vi "Send command to AutoCAD.vi"(4 "File name suffix":string, 5 "DesignRequest":T2, 6 "AC Variables":string[](array[string]), 7 "Mathcad Output":T3, 8 "error in (no error)":errorcluster, 9 "progress":refnum<vi>, 10 "Add":refnum<k24>, 11 "AutoCad app in":refnum<k24>) -> (0 "error out":errorcluster, 1 "progress out":refnum<vi>, 2 "Add out":refnum<k24>, 3 "AutoCad app out":refnum<k24>)   [LabVIEW 2012, in "Design Server.lvlib"]
uses:
  Design Server.lvlib
  Variable cluster.ctl
  Design Request.ctl
  C:/Program Files/Autodesk/AutoCAD 2013/Autodesk.AutoCAD.Interop.dll
  Program Files/Autodesk/AutoCAD 2013/Autodesk.AutoCAD.Interop.dll
panel:
  out "timing":T1
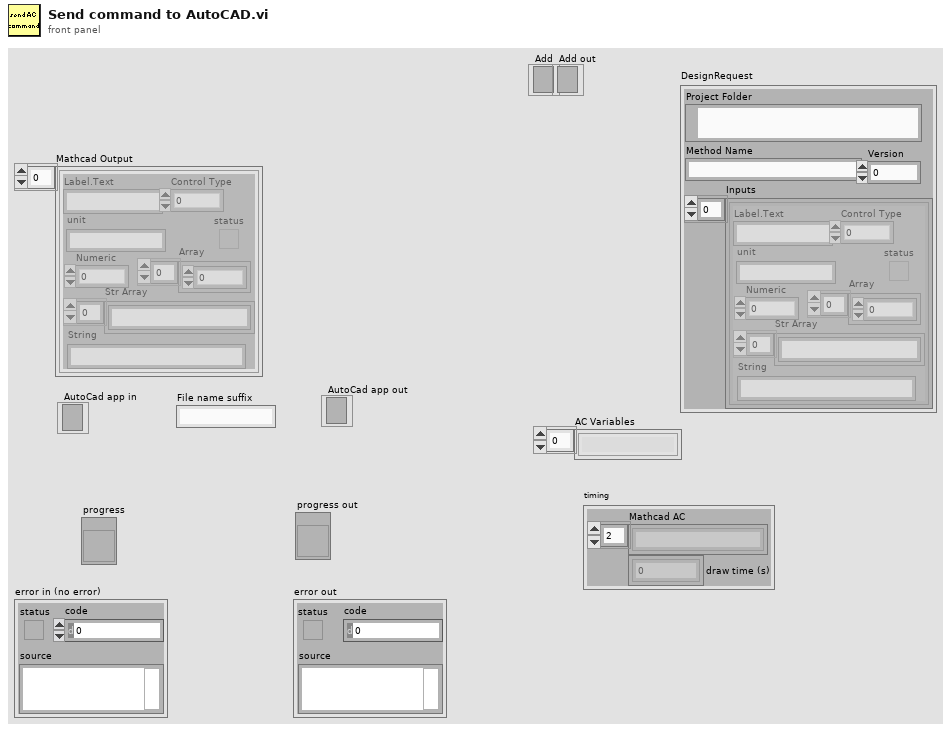
[diagram p1: front panel]
types:
  T1 = cluster{"draw time (s)":dbl[], "Mathcad AC":string[]}
  T2 = typedef "Design Server.lvlib/Design Request.ctl" = cluster{"Project Folder":path, "Method Name":string, "Inputs":T3, "Version":i32}
  T3 = typedef "Design Server.lvlib/Variable cluster.ctl" = cluster{"Label.Text":string, "Control Type":u32, "Numeric":dbl, "Array":dbl[], "status":bool, "Str Array":string[], "String":string, "unit":string}[]
  T4 = enum16{"open", "replace", "create", "open or create", "replace or create", "replace or create with confirmation"}
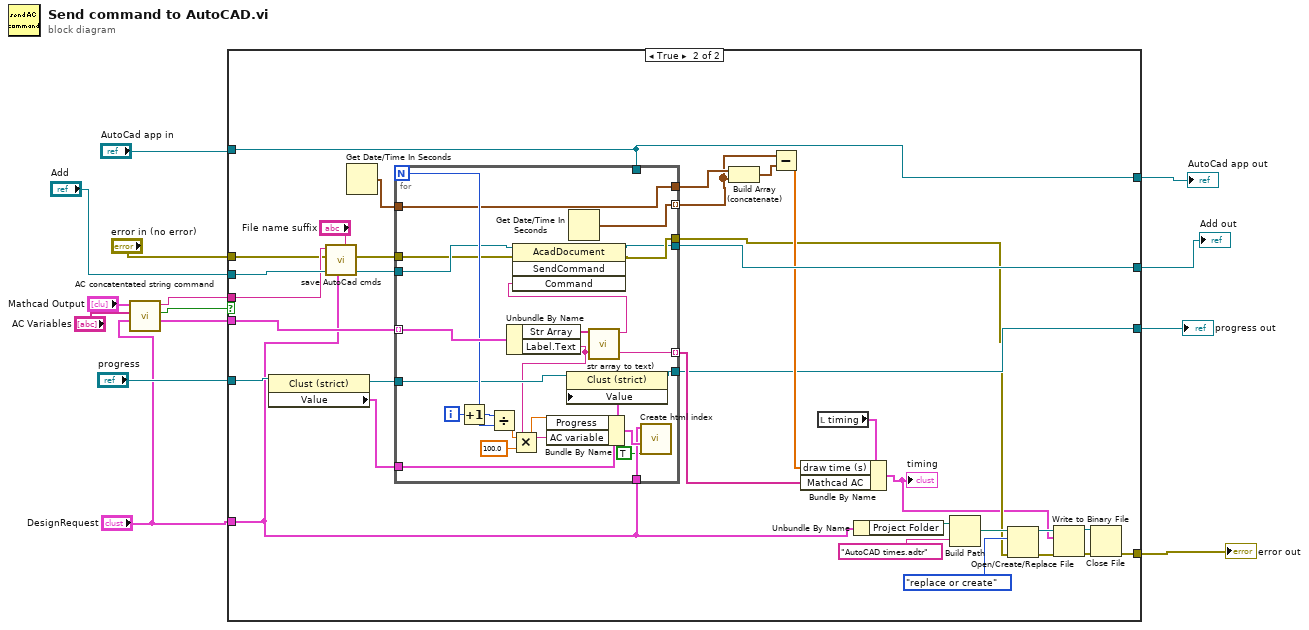
[diagram p0: block diagram]
diagram:
  n1 = call "AC concatentated string command.vi"("DesignRequest"="DesignRequest", "AC Variables"="AC Variables", "MathCAD results"="Mathcad Output") -> ("MathCAD AC"=w14:T3, "Has AC commands"=w8:bool, "AC concatenated string"=w6:string)  [unwired: 6 in]
  n2 = case shown="True" w8 {
    tunnel: w14 -> [_ w24]
    tunnel: [w18 w19] -> w3
    tunnel: "AutoCad app in" -> [w18 w19]
    tunnel: [w16 w48] -> w1
    tunnel: "Add" -> [w16 w47]
    tunnel: "error in (no error)" -> [w17 w21]
    tunnel: [w17 w34] -> w11
    tunnel: "progress" -> [w15 w30]
    tunnel: [w15 w29] -> w9
    tunnel: w6 -> [_ w25]
    tunnel: "DesignRequest" -> [_ w20]
    frame False {
    }
    frame True {
      n3 = property class="Clust (strict)"(reference=w30) -> (reference out=w49:refnum<vi>, "Value"=w42:cluster{"Progress":u8, "AC variable":string})  [unwired: 1 in, 1 out]
      n4 = call "save AutoCad cmds.vi"("File name suffix"="File name suffix", "DesignRequest"=w20, "error in"=w21, "AC.txt"=w25) -> ("error out"=w22:errorcluster)  [unwired: 7 in]
      n5 = Get Date/Time In Seconds() -> (seconds since 1Jan1904=w45:timestamp)
      n6 = for {
        N -> [w66]
        tunnel: w22 -> [w53]
        tunnel: w24 -> [w71] mode=indexing
        tunnel: w47 -> [w54]
        tunnel: [w50] -> w48
        tunnel: [w51] -> w28
        tunnel: w19 -> [_]
        tunnel: w49 -> [w61]
        tunnel: w42 -> [w70]
        tunnel: [w68] -> w29
        tunnel: [w55] -> w44 mode=indexing
        tunnel: [w60] -> w46
        tunnel: w45 -> [w60]
        tunnel: [w59] -> w40 mode=indexing
        tunnel: w20 -> [w57]
        i -> [w67]
        n7 = Increment(x=w67) -> (x+1=w62:i32)
        n8 = Divide(x=w62, y=w66) -> (x/y=w65:dbl)
        n9 = Unbundle By Name(w71) -> ("Str Array"=w69:string[], "Label.Text"=w59:string)
        n10 = Multiply(x=w65, y=100.0) -> (x*y=w63:dbl)
        n11 = Bundle By Name(cluster=w70, "Progress"=w63, "AC variable"=w59) -> (w58:cluster{"Progress":u8, "AC variable":string})
        n12 = property class="Clust (strict)"(reference=w61, "Value"=w58) -> (reference out=w68:refnum<vi>)  [unwired: 1 in, 1 out]
        n13 = Get Date/Time In Seconds() -> (seconds since 1Jan1904=w55:timestamp)
        n14 = call "str array to text).vi"("Array"=w69) -> ("String"=w52:string)  [unwired: 10 in]
        n15 = invoke class="AcadDocument" method="SendCommand"(reference=w54, error in=w53, "Command"=w52) -> (reference out=w50:refnum<k24>, error out=w51:errorcluster)  [unwired: 1 in, 2 out]
        n16 = call "Create html index.vi"("progress"=w58, "Under construction"=TRUE, "DesignRequest"=w57) -> ()  [unwired: 7 in, 2 out]
      }
      n17 = Build Array (concatenate)(w46, w44) -> (w43:timestamp[])
      n18 = Subtract(x=w44, y=w43) -> (x-y=w41:dbl[])
      n19 = local read "timing"() -> (w27:T1)
      n20 = Bundle By Name(cluster=w27, "draw time (s)"=w41, "Mathcad AC"=w40) -> (w26:T1)
      "timing" <- w26
      n21 = Unbundle By Name(w20) -> ("Project Folder"=w33:path)
      n22 = Build Path(base path=w33, name or relative path="AutoCAD times.adtr") -> (appended path=w31:path)
      n23 = Open/Create/Replace File(file path (use dialog)=w31, error in=w28, operation (0:open)=T4."replace or create") -> (refnum out=w37:refnum<file>, error out=w39:errorcluster)  [unwired: 3 in, 1 out]
      n24 = Write to Binary File(file (use dialog)=w37, data=w26, error in=w39) -> (refnum out=w35:refnum<file>, error out=w36:errorcluster)  [unwired: 3 in, 1 out]
      n25 = Close File(refnum=w35, error in=w36) -> (error out=w34:errorcluster)  [unwired: 1 out]
    }
  }
  "error out" <- w11
  "progress out" <- w9
  "AutoCad app out" <- w3
  "Add out" <- w1
